vi "GetAppOutput.vi"(8 "error in (no error)":errorcluster, 11 "LSEPlugin in":refnum<class "LSEPlugin.lvclass">) -> (0 "error out":errorcluster, 3 "LSEPlugin out":refnum<class "LSEPlugin.lvclass">)   [LabVIEW 2017, in "AppPlugins.lvlib" / "LSEPlugin.lvclass"]
uses:
  LSEPlugin.lvclass
  C:/dev/Work/PARTF/Modules/AppPlugins/AppPluginBaseClass/AppPluginsBase.lvclass
  Typedefs/LSEConfig.ctl
  AppPluginBaseClass/AppPluginsBase.lvclass/AppPluginsBase.ctl
  LSEPlugin.lvclass/LSEPlugin.ctl
  Typedefs/LSEOutput.ctl
  AppPluginBaseClass/Accessors/Read clEvtReportArray.vi
  Accessors/Read LSEConfig.vi
  <vilib>/Utility/error.llb/Error Cluster From Error Code.vi
  <vilib>/ErrorRing/Error Ring.xnode
panel:
  out "test_array":dbl[](array[numeric])
  out "Complete":bool
  out "LSEConfig":T1={"NoiseVariance"=0.0, "IEEESystem"=14, "PMULocations"=[0], "Vindex"=0, "Iindex"=3, "DynamicRef"=""}
  out "V_ang":dbl[][](array[numeric])
  out "V_mag":dbl[][](array[numeric])
  out "Number of PMUs":i32
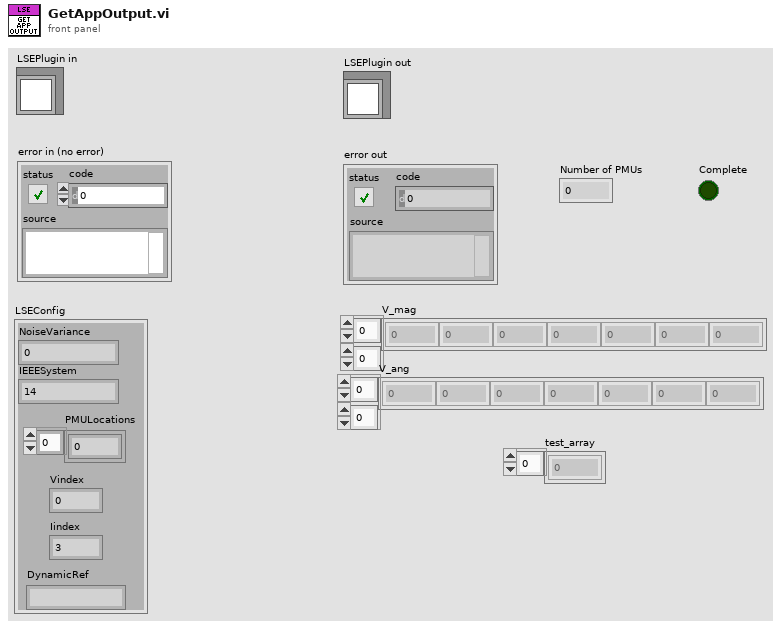
[diagram p1: front panel]
types:
  T1 = typedef "AppPlugins.lvlib/LSEPlugin.lvclass/LSEConfig.ctl" = cluster{"NoiseVariance":dbl, "IEEESystem":u32, "PMULocations":u32[], "Vindex":i32, "Iindex":i32, "DynamicRef":string}
  T2 = typedef "EventPlugins.lvlib/EventPluginBaseClass.lvclass/clEvtReportArray.ctl" = T3[]
  T3 = typedef "EventPlugins.lvlib/EventPluginBaseClass.lvclass/clEvtReport.ctl" = cluster{"Timestamp":dbl, "Synx":cdb[], "Freq":dbl, "ROCOF":dbl, "ID":i16}
  T4 = typedef "AppPlugins.lvlib/LSEPlugin.lvclass/Network.ctl" = cluster{"H":dbl[][], "Iij_num_vec":dbl[], "Iji_num_vec":dbl[], "Bus":dbl[], "PMUnumber":i32, "Iji_index":i32[]}
  T5 = typedef "AppPlugins.lvlib/LSEPlugin.lvclass/LSEOutput.ctl" = cluster{"SystemVoltagesRef":cdb[][], "Vestimate":cdb[][], "LSEConfig":T1, "Bus":dbl[]}
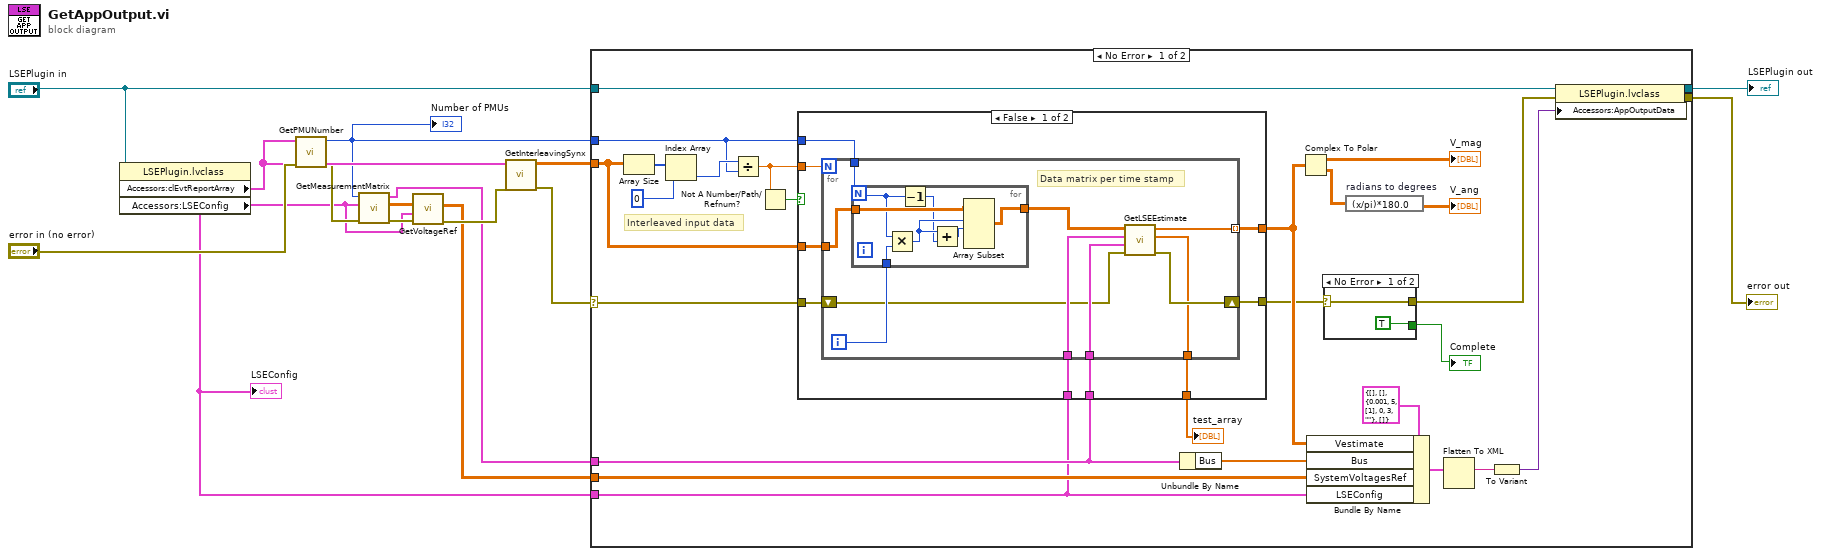
[diagram p0: block diagram]
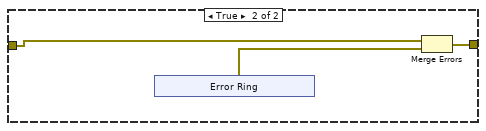
[diagram p2: hidden frame]
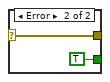
[diagram p3: hidden frame]
diagram:
  n1 = property class="LSEPlugin.lvclass"(reference="LSEPlugin in") -> ("Accessors:clEvtReportArray"=w12:T2, "Accessors:LSEConfig"=w2:T1)  [unwired: 1 in, 2 out]
  "LSEConfig" <- w2
  n2 = call "GetPMUNumber.vi"("error in (no error)"="error in (no error)", "Accessors:clEvtReportArray"=w12) -> ("error out"=w9:errorcluster, "size(s)"=w8:i32)  [unwired: 8 in]
  "Number of PMUs" <- w8
  n3 = call "GetMeasurementMatrix.vi"("error in"=w9, "lsecon"=w2, "PMUnumber"=w8) -> ("error out"=w7:errorcluster, "SystemVoltagesRef"=w3:cdb[][], "NetworkData"=w4:T4)  [unwired: 5 in]
  n4 = call "GetVoltageRef.vi"("error in (no error)"=w7, "lsecon"=w2, "SystemVoltagesRef"=w3) -> ("error out"=w6:errorcluster, "SystemVoltagesRef Out"=w5:cdb[][])  [unwired: 7 in]
  n5 = call "GetInterleavingSynx.vi"("error in (no error)"=w6, "clEvtReportArrayIn"=w12) -> ("error out"=w10:errorcluster, "Synx"=w11:cdb[][])  [unwired: 8 in]
  n6 = case shown="No Error" w10 {
    selector: w10 -> [w28 w81]
    tunnel: "LSEPlugin in" -> [w42 w82]
    tunnel: [w41 w82] -> w14
    tunnel: w11 -> [w29 _]
    tunnel: w8 -> [w27 _]
    tunnel: w5 -> [w25 _]
    tunnel: w4 -> [w24 _]
    tunnel: w2 -> [w23 _]
    tunnel: [w16 w81] -> w1
    frame No Error {
      # "Interleaved input data"
      n7 = Array Size(array=w29) -> (size(s)=w40:i32[])
      n8 = Index Array(array=w40, index=0) -> (element=w38:i32)
      n9 = Divide(x=w38, y=w27) -> (x/y=w21:dbl)
      n10 = Not A Number/Path/Refnum?(number/path/refnum=w21) -> (NaN/Path/Refnum?=w22:bool)
      n11 = case shown="False" w22 {
        tunnel: w21 -> [w51 _]
        tunnel: [w50 _] -> w34
        tunnel: [w49 w71] -> w32
        tunnel: w29 -> [w48 _]
        tunnel: w28 -> [w47 w69]
        tunnel: w27 -> [w46 _]
        tunnel: [w45 _] -> w26
        tunnel: w24 -> [w44 _]
        tunnel: w23 -> [w43 _]
        frame False {
          n12 = for {
            N: w51 -> [_]
            tunnel: w43 -> [w57]
            tunnel: [w52] -> w50 mode=indexing
            tunnel: w48 -> [w61]
            shift-right: [w54] -> w49
            shift-left: w47 -> [w55]
            tunnel: w44 -> [w56]
            tunnel: w46 -> [w59]
            tunnel: [w53] -> w45
            i -> [w60]
            # "Data matrix per time stamp"
            n13 = for {
              N: w59 -> [w65]
              tunnel: w61 -> [w68]
              tunnel: [w67] -> w58
              tunnel: w60 -> [w66]
              n14 = Multiply(x=w65, y=w66) -> (x*y=w64:i32)
              n15 = Decrement(x=w65) -> (x-1=w63:i32)
              n16 = Add(x=w64, y=w63) -> (x+y=w62:i32)
              n17 = Array Subset(array=w68, index (row)=w64, length (row)=w62) -> (w67:cdb[][])  [unwired: 2 in]
            }
            n18 = call "GetLSEEstimate.vi"("error in"=w55, "NetworkData"=w56, "lsecon"=w57, "measure_input"=w58) -> ("error out"=w54:errorcluster, "test_array"=w53:dbl[], "Vestimate"=w52:cdb[])  [unwired: 5 in]
          }
        }
        frame True {
          n19 = xnode "Error Ring"() -> ("error out"=w70:errorcluster)
          n20 = Merge Errors(w69, w70) -> (w71:errorcluster)
        }
      }
      "test_array" <- w26
      n21 = Unbundle By Name(w24) -> ("Bus"=w30:dbl[])
      n22 = Complex To Polar(r * e^(i*theta)=w34) -> (r=→"V_mag":dbl[][], theta=w36:dbl[][])
      n23 = Bundle By Name(cluster=T5 {"SystemVoltagesRef"=[], "Vestimate"=[], "LSEConfig"={"NoiseVariance"=0.001, "IEEESystem"=5, "PMULocations"=[1], "Vindex"=0, "Iindex"=3, "DynamicRef"=""}, "Bus"=[]} ("LSEOutput"), "Vestimate"=w34, "Bus"=w30, "SystemVoltagesRef"=w25, "LSEConfig"=w23) -> (w20:T5)
      n24 = case shown="No Error" w32 {
        selector: w32 -> [w78 w79]
        tunnel: [w78 w79] -> w17
        tunnel: [TRUE TRUE] -> w31
        frame No Error {
        }
        frame Error {
        }
      }
      "Complete" <- w31
      n25 = expression code="(x/pi)*180.0" "radians to degrees"(w36) -> (→"V_ang":dbl[][])
      n26 = Flatten To XML(anything=w20) -> (xml string=w19:string)
      n27 = To Variant(anything=w19) -> (Variant=w18:variant)
      n28 = property class="LSEPlugin.lvclass"(reference=w42, error in=w17, "Accessors:AppOutputData"=w18) -> (reference out=w41:refnum<class "LSEPlugin.lvclass">, error out=w16:errorcluster)
    }
    frame Error {
    }
  }
  "LSEPlugin out" <- w14
  "error out" <- w1
